vi "Close Event Handler.vi"(8 "error in (no error)":errorcluster, 11 "VolatusCore in":refnum<class "VolatusCore.lvclass">) -> (0 "error out":errorcluster, 3 "VolatusCore out":refnum<class "VolatusCore.lvclass">)   [LabVIEW 2020, in "Volatus.lvlib" / "VolatusCore.lvclass"]
uses:
  VolatusCore.lvclass
  VolatusCore.lvclass/VolatusCore.ctl
  Event API/EventAPI.lvclass
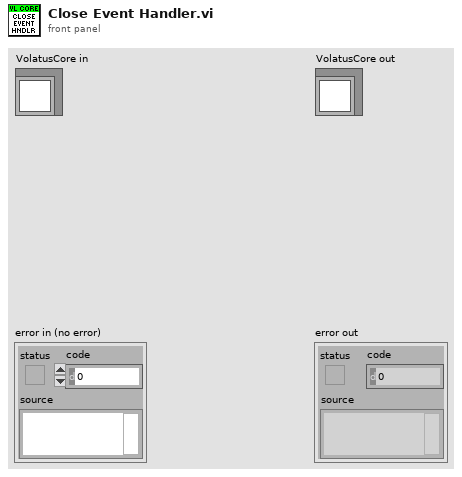
[diagram p1: front panel]
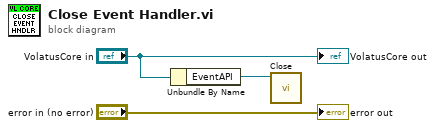
[diagram p0: block diagram]
diagram:
  n1 = Unbundle By Name("VolatusCore in") -> ("EventAPI"=w1:refnum<class "EventAPI.lvclass">)
  n2 = call "Close.vi"("EventAPI in"=w1) -> ()  [unwired: 9 in, 2 out]
  "error out" <- "error in (no error)"
  "VolatusCore out" <- "VolatusCore in"
